vi "Alert User to Failure.vi"(8 "error in (no error)":errorcluster, 11 "Failures":string) -> (0 "error out":errorcluster, 3 "Cancelled?":bool)   [LabVIEW 2015]
panel:
  in  "Cancel Button":bool
  in  "OK Button":bool
  # "Failure Conditions"
  # "The following failure conditions \nhave been found.\n\nPlease press OK to continue with\nthe test, or cancel to abort"
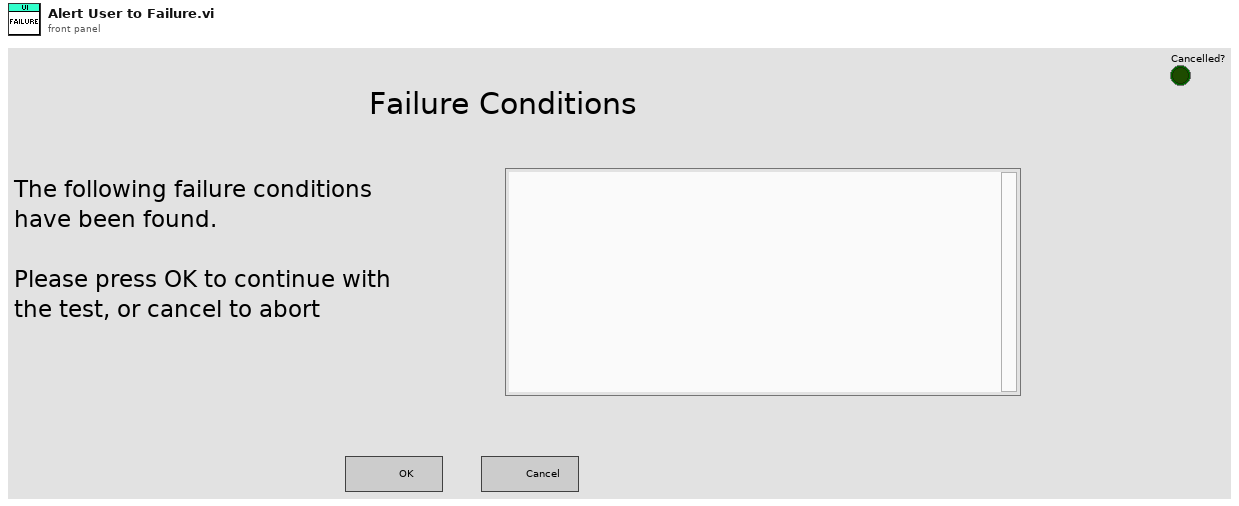
[diagram p1: front panel]
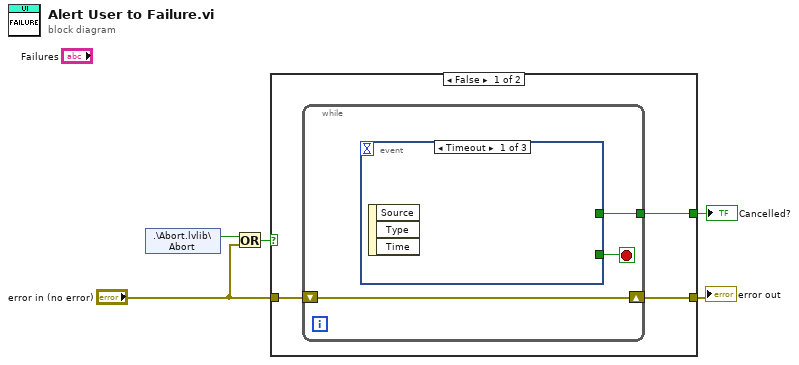
[diagram p0: block diagram]
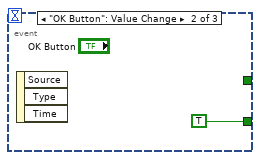
[diagram p2: hidden frame]
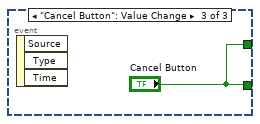
[diagram p3: hidden frame]
diagram:
  n1 = shared-variable ".\\Abort.lvlib\\Abort"() -> (w4:bool)  [unwired: 1 in, 1 out]
  n2 = Or(x=w4, y="error in (no error)") -> (x .or. y?=w3:bool)
  n3 = case shown="False" w3 {
    tunnel: [w8 w14] -> w5
    tunnel: "error in (no error)" -> [w7 w14]
    tunnel: [w6 _] -> w1
    frame False {
      n4 = while {
        shift-right: [w10] -> w8
        shift-left: w7 -> [w10]
        tunnel: [w9] -> w6
        stop <- w11 stop-if-true
        n5 = event shown="[0] Timeout" {
          selector: _ -> [_ _ _]
          dyn-events: _ -> [_ _ _]
          timeout: _ -> [_ _ _]
          tunnel: [_ TRUE "Cancel Button"] -> w11
          tunnel: [_ _ "Cancel Button"] -> w9
          event Timeout {
            n6 = event-data() -> ()  [unwired: 1 in, 3 out]
          }
          event "OK Button": Value Change {
            n7 = event-data() -> ()  [unwired: 1 in, 3 out]
          }
          event "Cancel Button": Value Change {
            n8 = event-data() -> ()  [unwired: 1 in, 3 out]
          }
        }
      }
    }
    frame True {
    }
  }
  "error out" <- w5
  "Cancelled?" <- w1
